vi "CreateSensorQueue.vi"(7 "ModuleID":i32, 8 "error in (no error)":errorcluster, 11 "AnalysisPluginsBase in":refnum<class "AnalysisPluginsBase.lvclass">) -> (0 "error out":errorcluster, 3 "AnalysisPluginsBase out":refnum<class "AnalysisPluginsBase.lvclass">)   [LabVIEW 2018, in "AnalysisPlugins.lvlib" / "AnalysisPluginsBase.lvclass"]
uses:
  AnalysisPluginsBase.lvclass
  Typedefs/clSensorData.ctl
  AnalysisPluginsBase.lvclass/AnalysisPluginsBase.ctl
  Accessors/Write SensorQue.vi
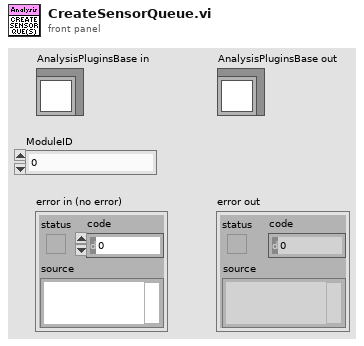
[diagram p1: front panel]
types:
  T1 = typedef "AnalysisPlugins.lvlib/AnalysisPluginsBase.lvclass/clSensorData.ctl" = cluster{"SensorType":string, "SensorData":variant, "TimeStamp":timestamp}
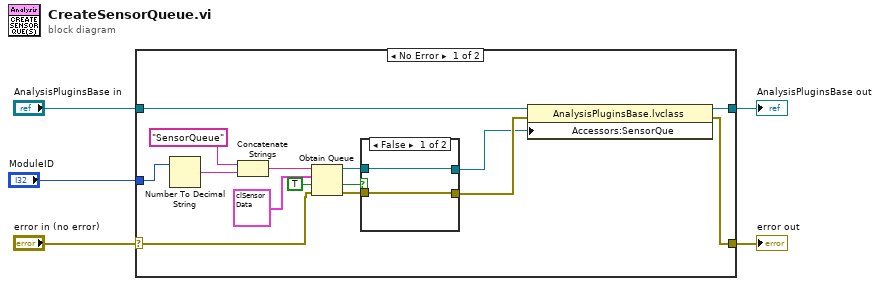
[diagram p0: block diagram]
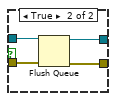
[diagram p2: hidden frame]
diagram:
  n1 = case shown="No Error" "error in (no error)" {
    selector: "error in (no error)" -> [w13 w28]
    tunnel: [w7 w28] -> w4
    tunnel: [w19 w27] -> w2
    tunnel: "AnalysisPluginsBase in" -> [w20 w27]
    tunnel: "ModuleID" -> [w6 _]
    frame No Error {
      n2 = Number To Decimal String(number=w6) -> (decimal integer string=w18:string)  [unwired: 1 in]
      n3 = Concatenate Strings("SensorQueue" ("string"), w18) -> (w16:string)
      n4 = Obtain Queue(name (unnamed)=w16, element data type=T1 {"SensorType"="", "SensorData"=variant, "TimeStamp"=timestamp(0 s since 1904-01-01)} ("clSensorData"), create if not found? (T)=TRUE, error in (no error)=w13) -> (queue out=w10:refnum<queue>, created new?=w12:bool, error out=w11:errorcluster)  [unwired: 1 in]
      n5 = case shown="False" w12 {
        tunnel: w11 -> [w21 w26]
        tunnel: w10 -> [w22 w25]
        tunnel: [w22 w24] -> w8
        tunnel: [w21 w23] -> w9
        frame False {
        }
        frame True {
          n6 = Flush Queue(queue=w25, error in (no error)=w26) -> (queue out=w24:refnum<queue>, error out=w23:errorcluster)  [unwired: 1 out]
        }
      }
      n7 = property class="AnalysisPluginsBase.lvclass"(reference=w20, error in=w9, "Accessors:SensorQue"=w8) -> (reference out=w19:refnum<class "AnalysisPluginsBase.lvclass">, error out=w7:errorcluster)
    }
    frame Error {
    }
  }
  "error out" <- w4
  "AnalysisPluginsBase out" <- w2
